vi "Get VISA gRPC Open Close Behavior.vi"(8 "error in (no error)":errorcluster, 11 "initialize session behavior":T2) -> (0 "error out":errorcluster, 3 "open/close behavior":T1)   [LabVIEW 2020, in "Keysight 34401A DMM Measurement.lvlib"]
uses:
  Keysight 34401A DMM Measurement.lvlib
  <vilib>/NI-VISA/VISA gRPC Open Close Behavior.ctl
  <vilib>/MeasurementLink/MeasurementLink Instrument/ISession Factory/Initialize and Close Session Behavior.ctl
  <vilib>/MeasurementLink/MeasurementLink Instrument/ISession Factory/ISession Factory.lvclass
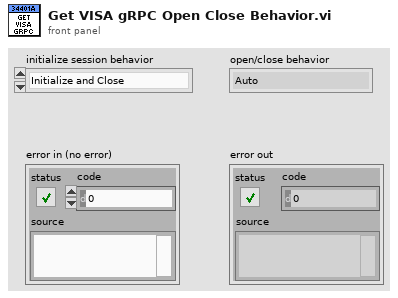
[diagram p1: front panel]
types:
  T1 = typedef "VISA gRPC Open Close Behavior.ctl" = enum16{"Auto", "Initialize and Close", "Attach and Detach", "Initialize and Detach", "Attach and Close"}
  T2 = typedef "MeasurementLink Instrument.lvlib/ISession Factory.lvclass/Initialize and Close Session Behavior.ctl" = enum16{"Initialize and Close", "Attach and Detach", "Initialize and Detach", "Attach and Close"}
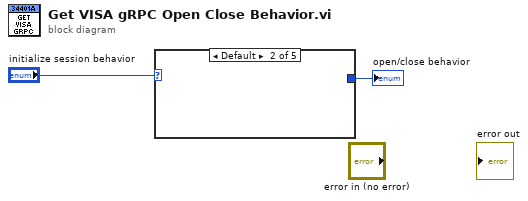
[diagram p0: block diagram]
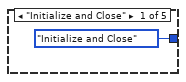
[diagram p2: hidden frame]
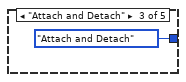
[diagram p3: hidden frame]
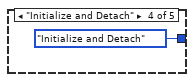
[diagram p4: hidden frame]
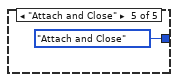
[diagram p5: hidden frame]
diagram:
  n1 = case shown="Default" "initialize session behavior" {
    tunnel: [VISA_gRPC_Open_Close_Behavior."Initialize and Close" ("open/close behavior") _ VISA_gRPC_Open_Close_Behavior."Attach and Detach" ("open/close behavior") VISA_gRPC_Open_Close_Behavior."Initialize and Detach" ("open/close behavior") VISA_gRPC_Open_Close_Behavior."Attach and Close" ("open/close behavior")] -> w1
    frame "Initialize and Close" {
    }
    frame Default {
    }
    frame "Attach and Detach" {
    }
    frame "Initialize and Detach" {
    }
    frame "Attach and Close" {
    }
  }
  "open/close behavior" <- w1
